vi "Q - not nan and gtr than zero - Real.vi"(8 "default":dbl, 10 "Numeric":dbl) -> (0 "out":dbl, 2 "Boolean":bool=TRUE)   [LabVIEW 2015]
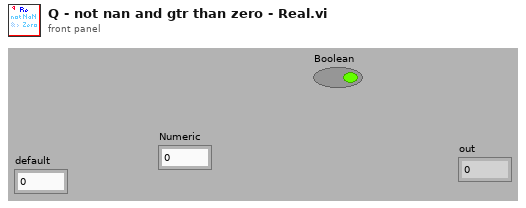
[diagram p1: front panel]
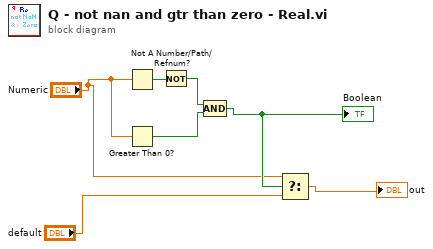
[diagram p0: block diagram]
diagram:
  n1 = Not A Number/Path/Refnum?(number/path/refnum="Numeric") -> (NaN/Path/Refnum?=w7:bool)
  n2 = Greater Than 0?(x="Numeric") -> (x > 0?=w6:bool)
  n3 = Not(x=w7) -> (.not. x?=w5:bool)
  n4 = Compound Arithmetic op=AND(w5, w6) -> (w4:bool)
  "Boolean" <- w4
  n5 = Select(t="Numeric", s=w4, f="default") -> (s? t:f=→"out":dbl)
